vi "18.2.-Conexión de VIs de Manera Remota (SLAVE).vi"() -> ()   [LabVIEW 2020]
panel:
  in  "stop":bool
  out "Waveform Chart":dbl(graph)
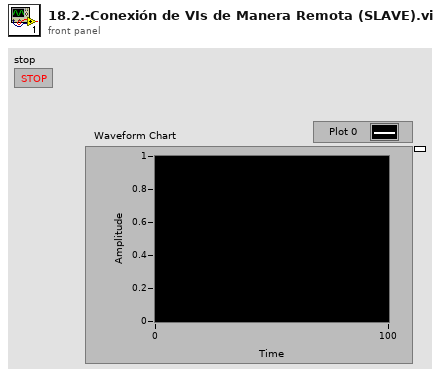
[diagram p1: front panel]
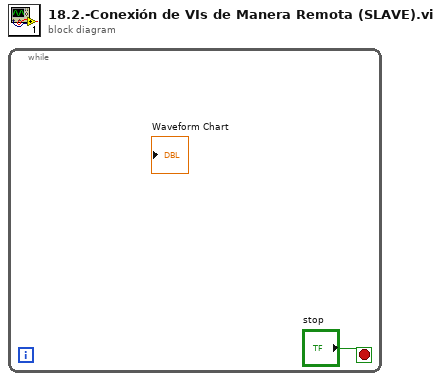
[diagram p0: block diagram]
diagram:
  n1 = while {
    stop <- "stop" stop-if-true
  }
